vi "Write Network Data to Optimization.vi"(7 "Network Data Array":T1[](array[typedef]), 8 "error in":errorcluster, 11 "Generic Optimization in":refnum<class "Generic Optimization.lvclass">) -> (0 "error out":errorcluster, 3 "Generic Optimization out":refnum<class "Generic Optimization.lvclass">)   [LabVIEW 2018, in "Generic Optimization Actor.lvlib" / "Generic Optimization.lvclass"]
uses:
  Generic Optimization.lvclass
  Optimization Controls/Electrical Network Optimization Data.ctl
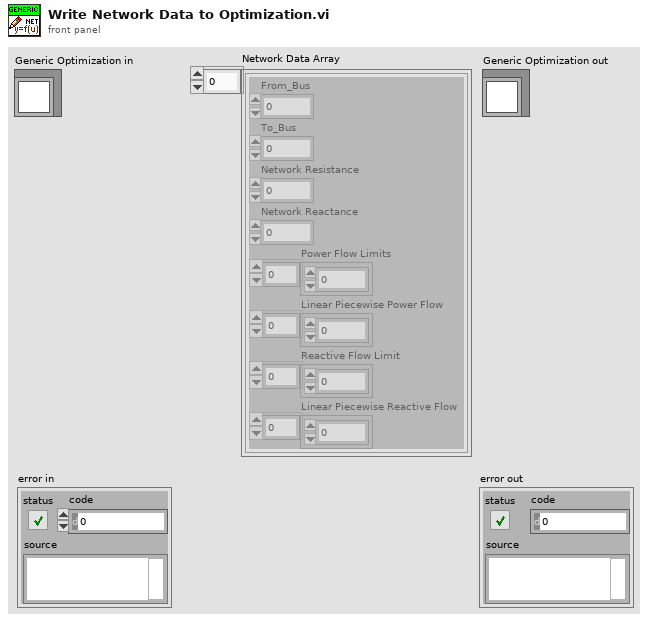
[diagram p1: front panel]
types:
  T1 = typedef "Generic Optimization Actor.lvlib/Generic Optimization.lvclass/Electrical Network Optimization Data.ctl" = cluster{"From_Bus":dbl, "To_Bus":dbl, "Network Resistance":dbl, "Network Reactance":dbl, "Power Flow Limits":dbl[], "Linear Piecewise Power Flow":dbl[], "Reactive Flow Limit":dbl[], "Linear Piecewise Reactive Flow":dbl[]}
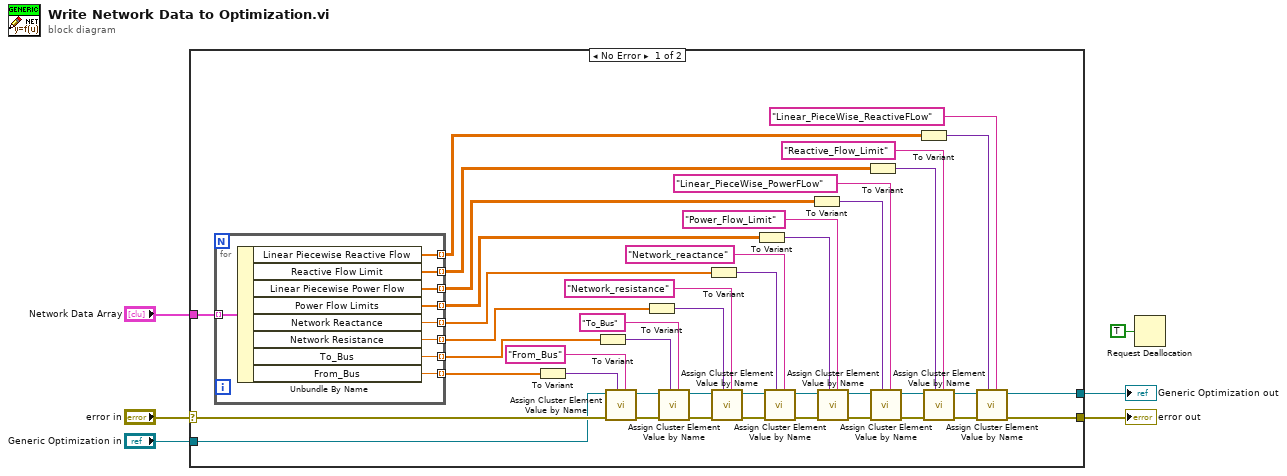
[diagram p0: block diagram]
diagram:
  n1 = case shown="No Error" "error in" {
    selector: "error in" -> [w28 w60]
    tunnel: [w49 w60] -> w6
    tunnel: "Network Data Array" -> [w17 _]
    tunnel: "Generic Optimization in" -> [w8 w59]
    tunnel: [w7 w59] -> w2
    frame No Error {
      n2 = for {
        tunnel: w17 -> [w58] mode=indexing
        tunnel: [w57] -> w9 mode=indexing
        tunnel: [w56] -> w10 mode=indexing
        tunnel: [w55] -> w11 mode=indexing
        tunnel: [w54] -> w12 mode=indexing
        tunnel: [w53] -> w13 mode=indexing
        tunnel: [w52] -> w14 mode=indexing
        tunnel: [w51] -> w15 mode=indexing
        tunnel: [w50] -> w16 mode=indexing
        n3 = Unbundle By Name(w58) -> ("Linear Piecewise Reactive Flow"=w57:dbl[], "Reactive Flow Limit"=w56:dbl[], "Linear Piecewise Power Flow"=w55:dbl[], "Power Flow Limits"=w54:dbl[], "Network Reactance"=w53:dbl, "Network Resistance"=w52:dbl, "To_Bus"=w51:dbl, "From_Bus"=w50:dbl)
      }
      n4 = To Variant(anything=w16) -> (Variant=w18:variant)
      n5 = To Variant(anything=w15) -> (Variant=w20:variant)
      n6 = call "Assign Cluster Element Value by Name.vi"("Element Name"="From_Bus" ("Keyword Name"), "Value"=w18, "error in"=w28, "Generic Optimization"=w8) -> ("error out"=w22:errorcluster, "Generic Optimization out"=w23:refnum<class "Generic Optimization.lvclass">)  [unwired: 6 in]
      n7 = To Variant(anything=w14) -> (Variant=w24:variant)
      n8 = call "Assign Cluster Element Value by Name.vi"("Element Name"="To_Bus" ("Keyword Name"), "Value"=w20, "error in"=w22, "Generic Optimization"=w23) -> ("error out"=w30:errorcluster, "Generic Optimization out"=w29:refnum<class "Generic Optimization.lvclass">)  [unwired: 6 in]
      n9 = To Variant(anything=w13) -> (Variant=w26:variant)
      n10 = call "Assign Cluster Element Value by Name.vi"("Element Name"="Network_resistance" ("Keyword Name"), "Value"=w24, "error in"=w30, "Generic Optimization"=w29) -> ("error out"=w32:errorcluster, "Generic Optimization out"=w31:refnum<class "Generic Optimization.lvclass">)  [unwired: 6 in]
      n11 = To Variant(anything=w12) -> (Variant=w33:variant)
      n12 = call "Assign Cluster Element Value by Name.vi"("Element Name"="Network_reactance" ("Keyword Name"), "Value"=w26, "error in"=w32, "Generic Optimization"=w31) -> ("error out"=w36:errorcluster, "Generic Optimization out"=w35:refnum<class "Generic Optimization.lvclass">)  [unwired: 6 in]
      n13 = To Variant(anything=w11) -> (Variant=w37:variant)
      n14 = call "Assign Cluster Element Value by Name.vi"("Element Name"="Power_Flow_Limit" ("Keyword Name"), "Value"=w33, "error in"=w36, "Generic Optimization"=w35) -> ("error out"=w44:errorcluster, "Generic Optimization out"=w43:refnum<class "Generic Optimization.lvclass">)  [unwired: 6 in]
      n15 = To Variant(anything=w10) -> (Variant=w39:variant)
      n16 = call "Assign Cluster Element Value by Name.vi"("Element Name"="Linear_PieceWise_PowerFLow" ("Keyword Name"), "Value"=w37, "error in"=w44, "Generic Optimization"=w43) -> ("error out"=w46:errorcluster, "Generic Optimization out"=w45:refnum<class "Generic Optimization.lvclass">)  [unwired: 6 in]
      n17 = To Variant(anything=w9) -> (Variant=w41:variant)
      n18 = call "Assign Cluster Element Value by Name.vi"("Element Name"="Reactive_Flow_Limit" ("Keyword Name"), "Value"=w39, "error in"=w46, "Generic Optimization"=w45) -> ("error out"=w48:errorcluster, "Generic Optimization out"=w47:refnum<class "Generic Optimization.lvclass">)  [unwired: 6 in]
      n19 = call "Assign Cluster Element Value by Name.vi"("Element Name"="Linear_PieceWise_ReactiveFLow" ("Keyword Name"), "Value"=w41, "error in"=w48, "Generic Optimization"=w47) -> ("error out"=w49:errorcluster, "Generic Optimization out"=w7:refnum<class "Generic Optimization.lvclass">)  [unwired: 6 in]
    }
    frame Error {
    }
  }
  "error out" <- w6
  "Generic Optimization out" <- w2
  n20 = Request Deallocation(TRUE ("flag")) -> ()
